vi "Write Binary Config.vi"(4 "Include Class Name":bool, 6 "byte order (0:big-endian, network order)":T1(ring), 8 "error in (no error)":errorcluster, 11 "AbsComp_Two Term_SGL in":refnum<class "AbsComp_Two Term_SGL.lvclass">) -> (0 "error out":errorcluster, 2 "Binary":string, 3 "AbsComp_Two Term_SGL out":refnum<class "AbsComp_Two Term_SGL.lvclass">)   [LabVIEW 2021, in "AbsComp_Two Term_SGL.lvclass"]
uses:
  AbsComp_Two Term_SGL.lvclass
  AbsComp_Two Term_SGL.lvclass/AbsComp_Two Term_SGL.ctl
  Abs_Types/Boolean/Abs_Boolean.lvclass
  Abs_Types/Single Float/Abs_Single Float.lvclass
  Abs_Types/Numeric/Abs_Numeric.lvclass
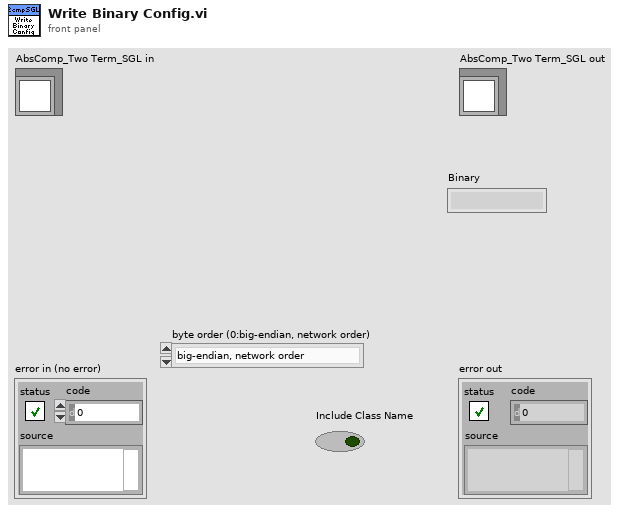
[diagram p1: front panel]
types:
  T1 = enum16{"big-endian, network order", "native, host order", "little-endian"}
  T2 = typedef "AbsComp_Two Term_SGL.lvclass/Abstract Type.ctl" = refnum<class "Abs_Single Float.lvclass">
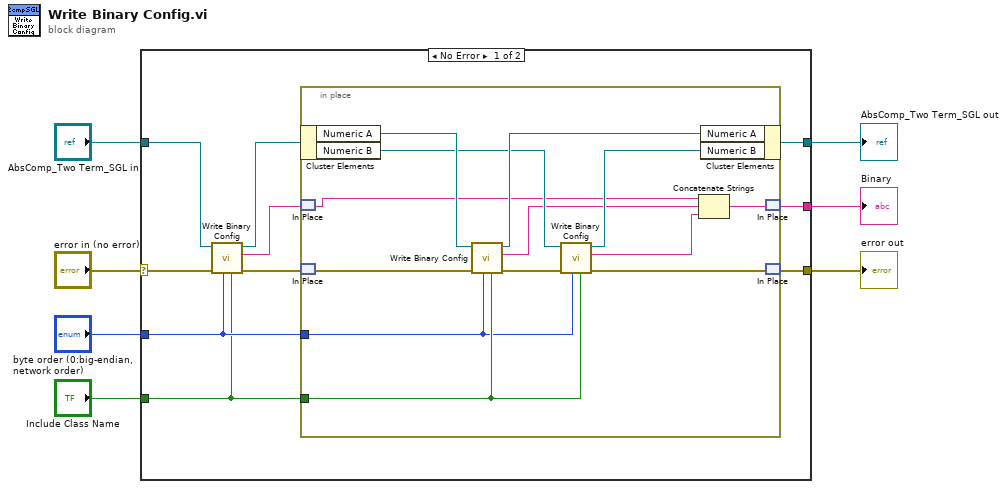
[diagram p0: block diagram]
diagram:
  n1 = case shown="No Error" "error in (no error)" {
    selector: "error in (no error)" -> [w17 w31]
    tunnel: "AbsComp_Two Term_SGL in" -> [w16 w32]
    tunnel: [w12 _] -> w2
    tunnel: "byte order (0:big-endian, network order)" -> [w11 _]
    tunnel: "Include Class Name" -> [w10 _]
    tunnel: [w9 w31] -> w3
    tunnel: [w8 w32] -> w1
    frame No Error {
      n2 = call-parent "Write Binary Config.vi"("Include Class Name"=w10, "byte order (0:big-endian, network order)"=w11, "error in (no error)"=w17, "Abs_Type in"=w16) -> ("error out"=w14:errorcluster, "Binary"=w13:string, "Abs_Type out"=w15:refnum<class "AbsComp_Two Term_SGL.lvclass">)  [unwired: 5 in]
      n3 = in-place {
        in-place-border: w11 -> [w21]
        in-place-border: w10 -> [w25]
        n4 = in-place-cluster #1(w15) -> ("Numeric A"=w28:T2, "Numeric B"=w27:refnum<class "Abs_Numeric.lvclass">)
        n5 = in-place-match #2(w13) -> (w20:string)
        n6 = in-place-match #3(w14) -> (w30:errorcluster)
        n7 = call-dynamic "Write Binary Config.vi"("Include Class Name"=w25, "byte order (0:big-endian, network order)"=w21, "error in (no error)"=w30, "Abs_Type in"=w28) -> ("error out"=w24:errorcluster, "Binary"=w19:string, "Abs_Type out"=w29:T2)  [unwired: 5 in]
        n8 = call-dynamic "Write Binary Config.vi"("Include Class Name"=w25, "byte order (0:big-endian, network order)"=w21, "error in (no error)"=w24, "Abs_Type in"=w27) -> ("error out"=w23:errorcluster, "Binary"=w22:string, "Abs_Type out"=w26:refnum<class "Abs_Numeric.lvclass">)  [unwired: 5 in]
        n9 = Concatenate Strings(w20, w19, w22) -> (w18:string)
        n10 = in-place-cluster #1("Numeric A"=w29, "Numeric B"=w26) -> (w8:refnum<class "AbsComp_Two Term_SGL.lvclass">)
        n11 = in-place-match #2(w18) -> (w12:string)
        n12 = in-place-match #3(w23) -> (w9:errorcluster)
      }
    }
    frame Error {
    }
  }
  "error out" <- w3
  "AbsComp_Two Term_SGL out" <- w1
  "Binary" <- w2
